vi "util.file.vars.file-operations.vi"(6 "allowDialogs?(False)":bool, 8 "error in (no error)":errorcluster, 9 "Operation(Read)":enum16{"Read File", "Write File"}(ring), 10 "selected path":path, 11 "Vars[] in":variant[](array[variant])) -> (0 "error out":errorcluster, 2 "filename":string, 3 "Procedure":variant[](array[variant]))   [LabVIEW 2024]
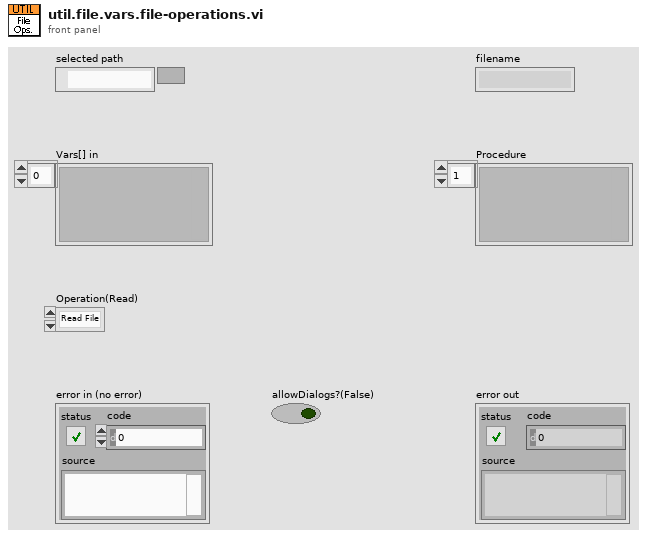
[diagram p1: front panel]
types:
  T1 = enum16{"open", "replace", "create", "open or create", "replace or create", "replace or create with confirmation"}
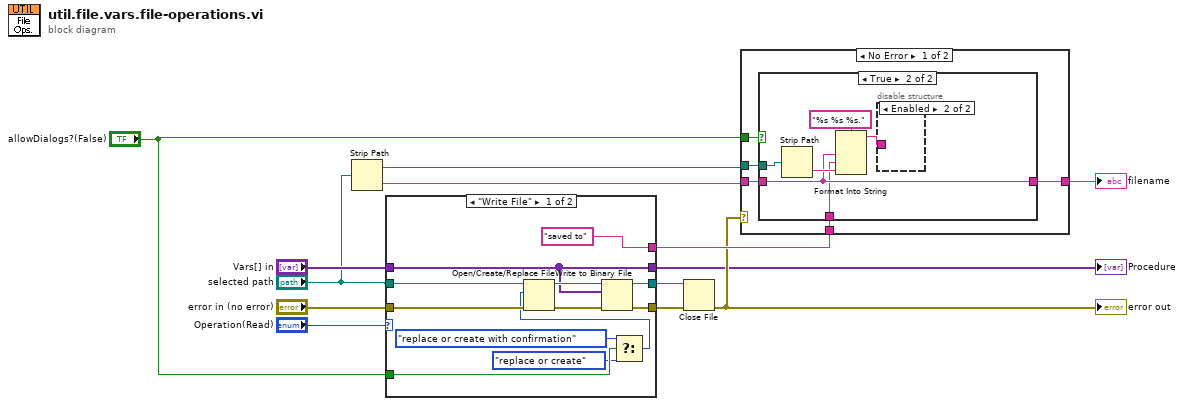
[diagram p0: block diagram]
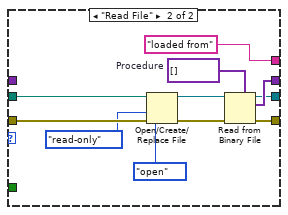
[diagram p2: hidden frame]
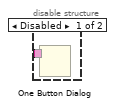
[diagram p4: hidden frame]
diagram:
  n1 = Strip Path(path="selected path") -> (stripped path=w8:path, name=w9:string)
  n2 = case shown="\"Write File\"" "Operation(Read)" {
    tunnel: [w14 w36] -> w2
    tunnel: "error in (no error)" -> [w23 w33]
    tunnel: [w22 w32] -> w4
    tunnel: [w21 w31] -> w5
    tunnel: "selected path" -> [w20 w29]
    tunnel: "allowDialogs?(False)" -> [w19 _]
    tunnel: ["saved to" ("name") "loaded from" ("name")] -> w12
    tunnel: "Vars[] in" -> [w14 _]
    frame "Write File" {
      n3 = Select(t=T1."replace or create with confirmation" ("operation (0:open)"), s=w19, f=T1."replace or create" ("operation (0:open)")) -> (s? t:f=w16:T1)
      n4 = Open/Create/Replace File(file path (use dialog)=w20, error in=w23, operation (0:open)=w16) -> (refnum out=w25:refnum<file>, error out=w24:errorcluster)  [unwired: 3 in, 1 out]
      n5 = Write to Binary File(file (use dialog)=w25, data=w14, error in=w24) -> (refnum out=w22:refnum<file>, error out=w21:errorcluster)  [unwired: 3 in, 1 out]
    }
    frame "Read File" {
      w30 = variant[] []  # Procedure
      n6 = Open/Create/Replace File(file path (use dialog)=w29, error in=w33, operation (0:open)=T1."open", access (0:read/write)=enum16{"read/write", "read-only", "write-only"}."read-only") -> (refnum out=w35:refnum<file>, error out=w34:errorcluster)  [unwired: 2 in, 1 out]
      n7 = Read from Binary File(5:w30, 8:w34, 11:w35) -> (0:w31:errorcluster, 2:w36:variant[], 3:w32:refnum<file>)  [unwired: 3 in, 1 out]
    }
  }
  "Procedure" <- w2
  n8 = Close File(refnum=w4, error in=w5) -> (error out=w6:errorcluster)  [unwired: 1 out]
  "error out" <- w6
  n9 = case shown="No Error" w6 {
    tunnel: "allowDialogs?(False)" -> [w41 _]
    tunnel: w8 -> [w40 _]
    tunnel: w9 -> [w39 w50]
    tunnel: [w38 w50] -> w10
    tunnel: w12 -> [w37 _]
    frame No Error {
      n10 = case shown="True" w41 {
        tunnel: w40 -> [_ w45]
        tunnel: w39 -> [w42 w44]
        tunnel: [w42 w44] -> w38
        tunnel: w37 -> [_ w43]
        frame False {
        }
        frame True {
          n11 = Strip Path(path=w45) -> (name=w48:string)  [unwired: 1 out]
          n12 = Format Into String(format string="%s %s %s.", w44, w43, w48) -> (resulting string=w46:string)  [unwired: 2 in, 1 out]
          n13 = disable-structure shown="Enabled" {
            disable-tunnel: w46 -> [w49 _]
            frame Disabled {
              n14 = One Button Dialog(message=w49) -> ()  [unwired: 1 in, 1 out]
            }
            frame Enabled {
            }
          }
        }
      }
    }
    frame Error {
    }
  }
  "filename" <- w10
